vi "BME_DG_LoadCardParameters.vi"(7 "DG_Number":i32, 8 "error in (no error)":errorcluster, 9 "TimeList":bool, 10 "ModuloCounter":bool, 11 "EventCounter":bool) -> (0 "error out":errorcluster)   [LabVIEW 2009, in "POLARIS BME DG.lvlib"]
uses:
  POLARIS BME DG.lvlib
  BME DLL/DelayGenerator.dll
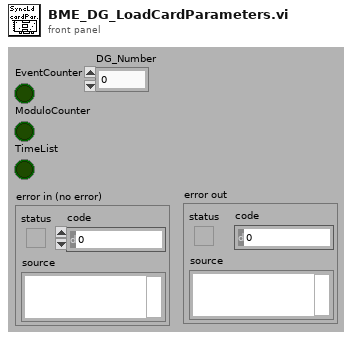
[diagram p1: front panel]
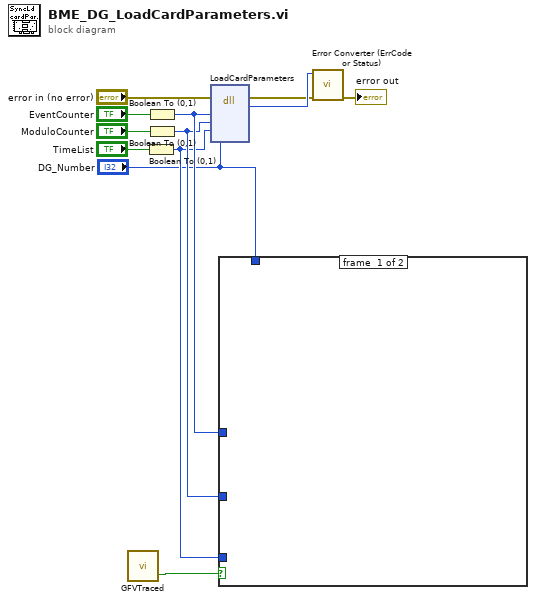
[diagram p0: block diagram]
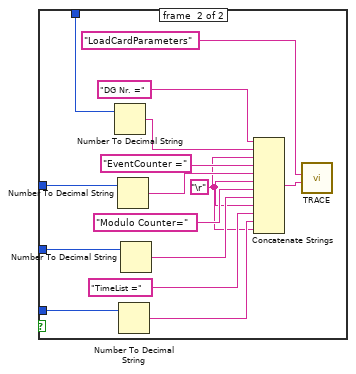
[diagram p2: hidden frame]
diagram:
  n1 = call "GFVTraced.vi"() -> ("traced?"=w5:bool)  [unwired: 2 in]
  n2 = Boolean To (0,1)(Boolean="TimeList") -> (0, 1=w2:i16)
  n3 = Boolean To (0,1)(Boolean="EventCounter") -> (0, 1=w4:i16)
  n4 = Boolean To (0,1)(Boolean="ModuloCounter") -> (0, 1=w3:i16)
  n5 = dll-call lib="D:/CS Framework/LVSCC/LV2009/GPL/Projects/cs-framework/CSClass/CSPOLARIS/POLARIS BME DG/BME DLL/DelayGenerator.dll" fn="LoadCardParameters"(error in="error in (no error)", "bEventCounter"=w4, "bModuloCounter"=w3, "bTimeList"=w2, "DG#"="DG_Number") -> (error out=w10:errorcluster, "return type"=w11:i32)  [unwired: 6 in, 1 out]
  n6 = case shown="True" w5 {
    tunnel: w4 -> [_ w24]
    tunnel: w3 -> [_ w19]
    tunnel: w2 -> [_ w17]
    tunnel: "DG_Number" -> [_ w13]
    frame #0 {
    }
    frame #1 {
      w16 = "\r"
      n7 = Number To Decimal String(number=w13) -> (decimal integer string=w14:string)  [unwired: 1 in]
      n8 = Number To Decimal String(number=w24) -> (decimal integer string=w23:string)  [unwired: 1 in]
      n9 = Number To Decimal String(number=w17) -> (decimal integer string=w18:string)  [unwired: 1 in]
      n10 = Number To Decimal String(number=w19) -> (decimal integer string=w21:string)  [unwired: 1 in]
      n11 = Concatenate Strings("DG Nr. =", w14, w16, "EventCounter =", w23, w16, "Modulo Counter=", w21, w16, "TimeList =", w18, w16) -> (w25:string)
      n12 = call "TRACE.vi"("Parameter String"=w25, "Function"="LoadCardParameters") -> ()  [unwired: 10 in]
    }
  }
  n13 = call "Error Converter (ErrCode or Status).vi"("error in (no error)"=w10, "error code"=w11) -> ("error out"=→"error out":errorcluster)  [unwired: 9 in]
